vi "get enum reference.vi"(8 "error in":errorcluster, 11 "displayable in":refnum<class "displayable.lvclass">) -> (0 "error out":errorcluster, 2 "enum":variant, 3 "displayable out":refnum<class "displayable.lvclass">)   [LabVIEW 2013, in "displayable.lvclass"]
uses:
  displayable.lvclass
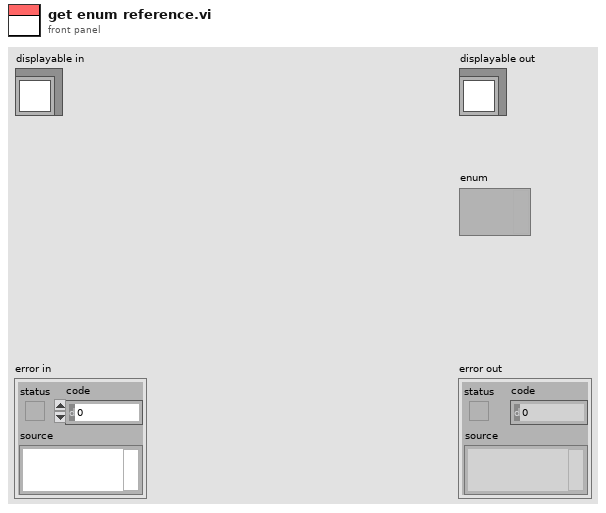
[diagram p1: front panel]
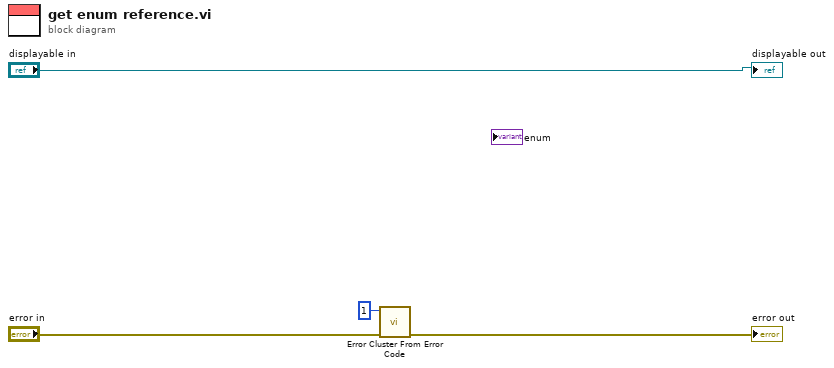
[diagram p0: block diagram]
diagram:
  n1 = call <vilib>:"Error Cluster From Error Code.vi"("error in (no error)"="error in", "error code (0)"=1) -> ("error out"=→"error out":errorcluster)  [unwired: 7 in]
  "displayable out" <- "displayable in"
